vi "Read serialNumber.vi"(8 "error in (no error)":errorcluster, 11 "Monochromator in":refnum<class "Monochromator.lvclass">) -> (0 "error out":errorcluster, 2 "serialNumber":string, 3 "Monochromator out":refnum<class "Monochromator.lvclass">)   [LabVIEW 2023, in "Monochromator.lvclass"]
doc: "Accessor VI for this class property."
uses:
  Monochromator.lvclass
  GenericDevice/GenericDevice.lvclass
panel:
  # "Connector Pane"
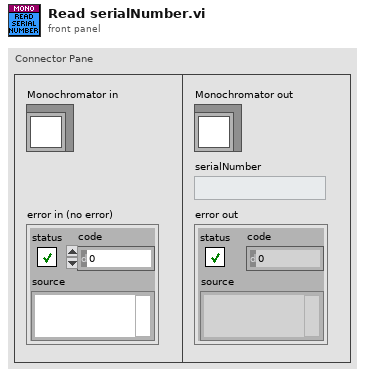
[diagram p1: front panel]
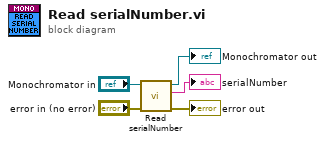
[diagram p0: block diagram]
diagram:
  n1 = call-parent "Read serialNumber.vi"("error in (no error)"="error in (no error)", "GenericDevice in"="Monochromator in") -> ("error out"=→"error out":errorcluster, "serialNumber"=→"serialNumber":string, "GenericDevice out"=→"Monochromator out":refnum<class "Monochromator.lvclass">)  [unwired: 7 in]
